vi "config not UI to UI (AO and AI).vi"(8 "error in (no error)":errorcluster, 10 "AO Config":T9 {"terminal configuration" items=[""=-1, "differential"=10106, "pseudodifferential"=12529]}, 11 "AI Config":T7 {"terminal configuration" items=[""=-1, "differential"=10106, "pseudodifferential"=12529]; "Coupling" items=[""=0, "AC"=10045, "DC"=10050, "GND"=10066]}) -> (0 "error out":errorcluster, 3 "New Ch []":T1 {"AI terminal config" items=[""=-1, "differential"=10106, "pseudodifferential"=12529]; "AI.Coupling" items=[""=0, "AC"=10045, "DC"=10050, "GND"=10066]; "AO terminal config" items=[""=-1, "differential"=10106, "pseudodifferential"=12529]})   [LabVIEW 2019, in "Instrument.Lockin.lvlib" / "Instrument.Lockin.lvclass"]
uses:
  Instrument.Lockin.lvclass
  Instrument.DAQ/Typedefs/DAQ.Config.AO--Cluster--Array.ctl
  Instrument.DAQ/Typedefs/DAQ.Config.AO.Range--enum.ctl
  Instrument.DAQ/Typedefs/DAQ.TerminalConfiguration--ring.ctl
  Instrument.DAQ/Typedefs/DAQ.Type--enum.ctl
  Instrument.DAQ/Typedefs/DAQ.Config.AI--Cluster--Array.ctl
  Instrument.DAQ/Typedefs/DAQ.Config.AI.Coupling--enum.ctl
  Instrument.DAQ/Typedefs/DAQ.Config.AI.Range--enum.ctl
  Instrument.DAQ/Typedefs/DAQ.Configuration--Cluster--Array.ctl
  Instrument.DAQ/Typedefs/DAQ.Configuration--Cluster.ctl
  Instrument.DAQ/Instrument.DAQ.lvclass
panel:
  # "Device"
  # "AI.Ch"
  # "AI.Range"
  # "AI.Coupling"
  # "AO.Ch"
  # "AO.Range"
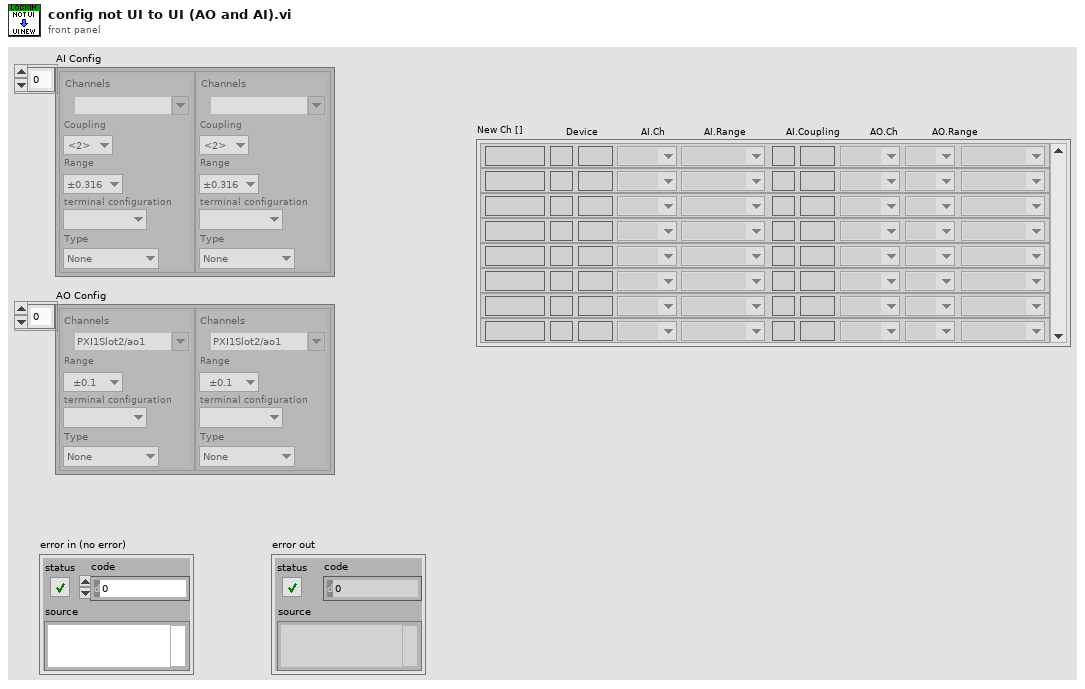
[diagram p1: front panel]
types:
  T1 = typedef "Instrument.Lockin.lvlib/Instrument.DAQ.lvclass/DAQ.Configuration--Cluster--Array.ctl" = T2[]
  T2 = typedef "Instrument.Lockin.lvlib/Instrument.DAQ.lvclass/DAQ.Configuration--Cluster.ctl" = cluster{"Device":string, "Lockin.AO":string, "AO.Ch":string, "AO.Range":T3, "AO terminal config":T4, "Lockin.AI":string, "AI.Ch":string, "AI.Range":T5, "AI.Coupling":T6, "AI terminal config":T4}
  T3 = typedef "Instrument.Lockin.lvlib/Instrument.DAQ.lvclass/DAQ.Config.AO.Range--enum.ctl" = enum16{"±0.1", "±1.0", "±3.5", "±10.0", ""}
  T4 = typedef "Instrument.Lockin.lvlib/Instrument.DAQ.lvclass/DAQ.TerminalConfiguration--ring.ctl" = i32
  T5 = typedef "Instrument.Lockin.lvlib/Instrument.DAQ.lvclass/DAQ.Config.AI.Range--enum.ctl" = enum16{"±0.316", "±1.00", "±3.16", "±10.0", "±31.6", "±42.4", ""}
  T6 = typedef "Instrument.Lockin.lvlib/Instrument.DAQ.lvclass/DAQ.Config.AI.Coupling--enum.ctl" = u16
  T7 = typedef "Instrument.Lockin.lvlib/Instrument.DAQ.lvclass/DAQ.Config.AI--Cluster--Array.ctl" = cluster{"Channels":tag, "Coupling":T6, "Range":T5, "terminal configuration":T4, "Type":T8}[]
  T8 = typedef "Instrument.Lockin.lvlib/Instrument.DAQ.lvclass/DAQ.Type--enum.ctl" = enum16{"None", "USB-4431", "PXI-446x"}
  T9 = typedef "Instrument.Lockin.lvlib/Instrument.DAQ.lvclass/DAQ.Config.AO--Cluster--Array.ctl" = cluster{"Channels":tag, "Range":T3, "terminal configuration":T4, "Type":T8}[]
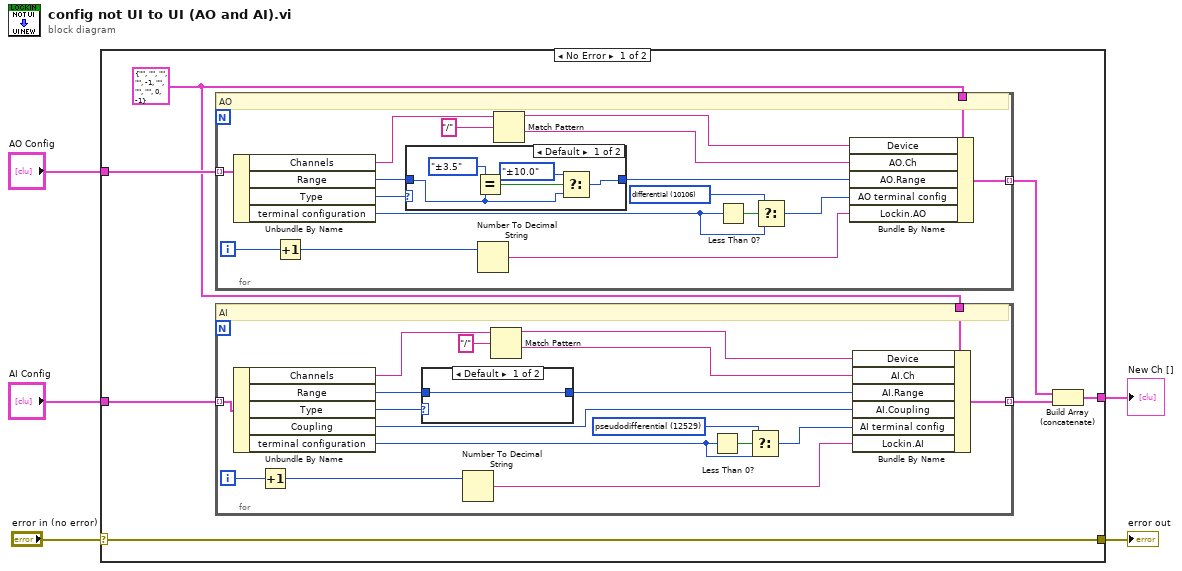
[diagram p0: block diagram]
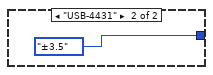
[diagram p2: hidden frame]
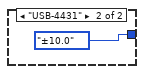
[diagram p3: hidden frame]
diagram:
  n1 = case shown="No Error" "error in (no error)" {
    selector: "error in (no error)" -> [w12 w56]
    tunnel: "AO Config" -> [w10 _]
    tunnel: [w9 _] -> w2
    tunnel: [w12 w56] -> w3
    tunnel: "AI Config" -> [w11 _]
    frame No Error {
      w6 = T2 {"Device"="", "Lockin.AO"="", "AO.Ch"="", "AO.Range"=enum."", "AO terminal config"=-1, "Lockin.AI"="", "AI.Ch"="", "AI.Range"=enum."", "AI.Coupling"=0, "AI terminal config"=-1} ("DAQ.Config")
      n2 = for {
        tunnel: w10 -> [w29] mode=indexing
        tunnel: [w25] -> w8 mode=indexing
        tunnel: w6 -> [w24]
        i -> [w18]
        w22 = T4 10106 items=[""=-1, "differential"=10106, "pseudodifferential"=12529] ("terminal configuration")
        # "AO"
        n3 = Unbundle By Name(w29) -> ("Channels"=w15:tag, "Range"=w13:T3, "Type"=w14:T8, "terminal configuration"=w21:T4)
        n4 = Increment(x=w18) -> (x+1=w19:i32)
        n5 = case shown="Default" w14 {
          tunnel: [w32 DAQ.Config.AO.Range--enum."±3.5" ("AO.Range")] -> w16
          tunnel: w13 -> [w30 _]
          frame Default {
            n6 = Equal?(x=DAQ.Config.AO.Range--enum."±3.5" ("AO.Range"), y=w30) -> (x = y?=w34:bool)
            n7 = Select(t=DAQ.Config.AO.Range--enum."±10.0" ("AO.Range"), s=w34, f=w30) -> (s? t:f=w32:T3)
          }
          frame "USB-4431" {
          }
        }
        n8 = Number To Decimal String(number=w19) -> (decimal integer string=w17:string)  [unwired: 1 in]
        n9 = Match Pattern(string=w15, regular expression="/") -> (before substring=w27:string, after substring=w26:string)  [unwired: 1 in, 2 out]
        n10 = Less Than 0?(x=w21) -> (x < 0?=w23:bool)
        n11 = Select(t=w22, s=w23, f=w21) -> (s? t:f=w20:T4)
        n12 = Bundle By Name(cluster=w24, "Device"=w27, "AO.Ch"=w26, "AO.Range"=w16, "AO terminal config"=w20, "Lockin.AO"=w17) -> (w25:T2)
      }
      n13 = for {
        tunnel: [w53] -> w7 mode=indexing
        tunnel: w6 -> [w52]
        tunnel: w11 -> [w51] mode=indexing
        i -> [w44]
        w46 = T4 12529 items=[""=-1, "differential"=10106, "pseudodifferential"=12529] ("terminal configuration")
        # "AI"
        n14 = Unbundle By Name(w51) -> ("Channels"=w40:tag, "Range"=w36:T5, "Type"=w41:T8, "Coupling"=w38:T6, "terminal configuration"=w42:T4)
        n15 = Increment(x=w44) -> (x+1=w45:i32)
        n16 = case shown="Default" w41 {
          tunnel: [w54 DAQ.Config.AI.Range--enum."±10.0" ("AI.Range")] -> w37
          tunnel: w36 -> [w54 _]
          frame Default {
          }
          frame "USB-4431" {
          }
        }
        n17 = Number To Decimal String(number=w45) -> (decimal integer string=w43:string)  [unwired: 1 in]
        n18 = Match Pattern(string=w40, regular expression="/") -> (before substring=w39:string, after substring=w49:string)  [unwired: 1 in, 2 out]
        n19 = Less Than 0?(x=w42) -> (x < 0?=w48:bool)
        n20 = Select(t=w46, s=w48, f=w42) -> (s? t:f=w47:T4)
        n21 = Bundle By Name(cluster=w52, "Device"=w39, "AI.Ch"=w49, "AI.Range"=w37, "AI.Coupling"=w38, "AI terminal config"=w47, "Lockin.AI"=w43) -> (w53:T2)
      }
      n22 = Build Array (concatenate)(w8, w7) -> (w9:T2[])
    }
    frame Error {
    }
  }
  "error out" <- w3
  "New Ch []" <- w2
